vi "op_theremin_main.vi"() -> ()   [LabVIEW 2018]
uses:
  op_theremin_state_defining_enum.ctl
  sig_processing_state_defining_enum.ctl
panel:
  in  "Frequency 2":dbl(knob) min=0.0 max=20000.0 scale=0.0..20000.0
  in  "Frequency":dbl(knob) min=0.0 max=20000.0 scale=0.0..20000.0
  in  "Vertical Pointer Slide":dbl(slide) scale=0.0..10.0
  in  "Frequency":dbl(slide)=20.0 min=0.0 max=20000.0 scale=0.0..20000.0
  in  "Stop":bool
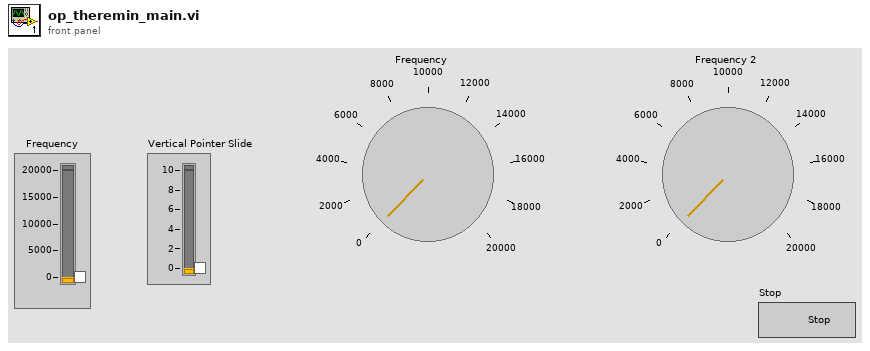
[diagram p1: front panel]
types:
  T1 = typedef "op_theremin_state_defining_enum.ctl" = enum16{"INIT", "SHDN", "RUN"}
  T2 = typedef "sig_processing_state_defining_enum.ctl" = enum16{"Coerce", "Scale", "Offset", "Norm"}
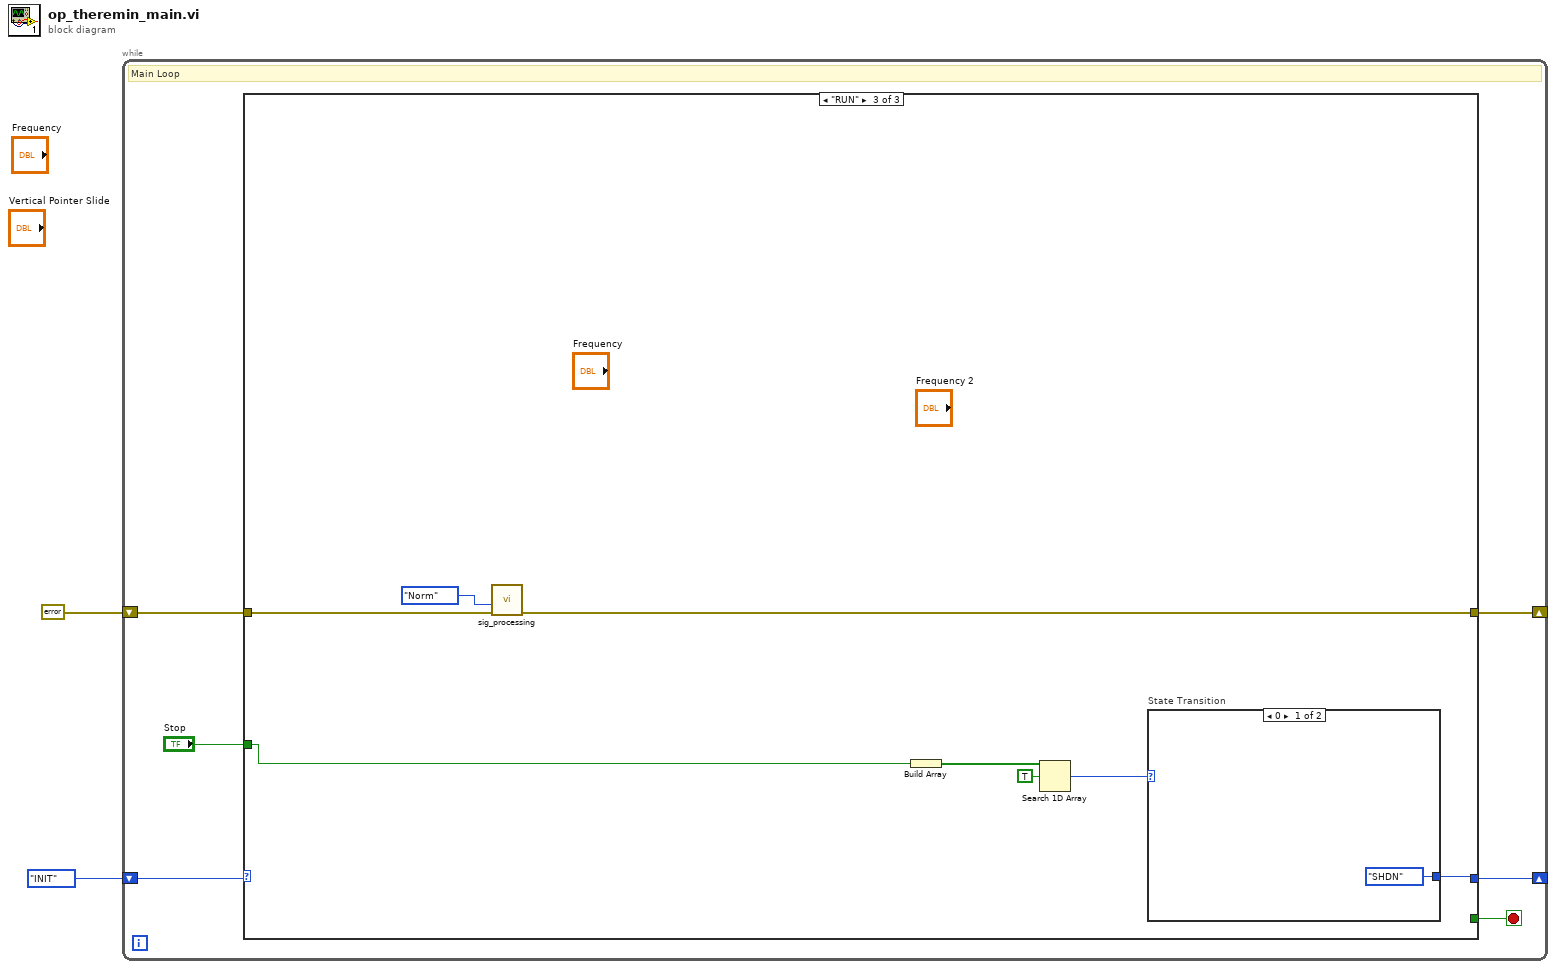
[diagram p0: block diagram]
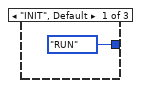
[diagram p2: hidden frame]
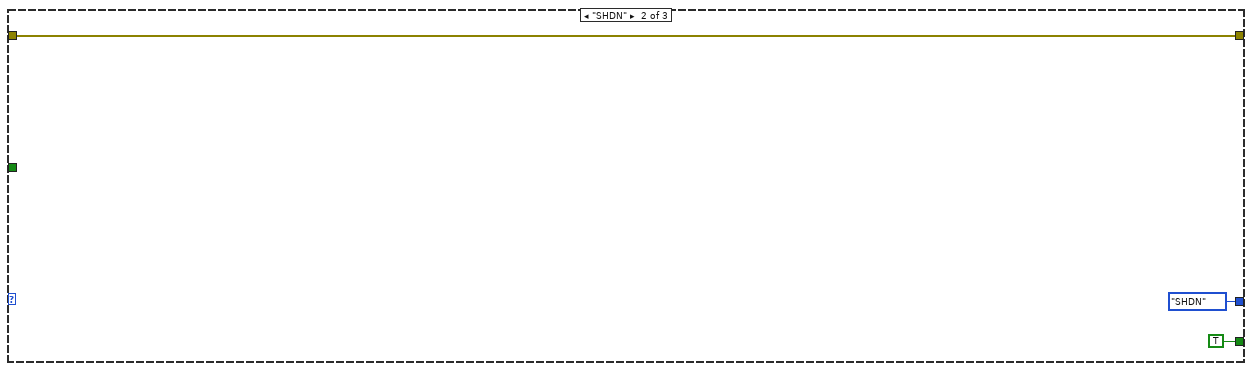
[diagram p3: hidden frame]
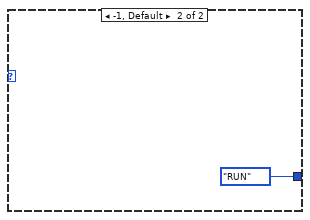
[diagram p4: hidden frame]
diagram:
  n1 = while {
    shift-right: [w6] -> _
    shift-left: op_theremin_state_defining_enum."INIT" -> [w7]
    shift-right: [w3] -> _
    shift-left: errorcluster {"status"=FALSE, "code"=0, "source"=""} ("error constant") -> [w4]
    stop <- w8 stop-if-true
    # "Main Loop"
    n2 = case shown="\"RUN\"" w7 {
      tunnel: [_ TRUE _] -> w8
      tunnel: [op_theremin_state_defining_enum."RUN" op_theremin_state_defining_enum."SHDN" w18] -> w6
      tunnel: "Stop" -> [_ _ w17]
      tunnel: w4 -> [_ w11 w15]
      tunnel: [_ w11 w14] -> w3
      frame "INIT", Default {
      }
      frame "SHDN" {
      }
      frame "RUN" {
        n3 = call "sig_processing.vi"("error in (no error)"=w15, "Operation"=sig_processing_state_defining_enum."Norm") -> ("error out"=w14:errorcluster)  [unwired: 8 in, 1 out]
        n4 = Build Array(w17) -> (w16:bool[])
        n5 = Search 1D Array(1D array=w16, element=TRUE) -> (index of element=w19:i32)  [unwired: 1 in]
        n6 = case "State Transition" shown="0" w19 {
          tunnel: [op_theremin_state_defining_enum."SHDN" op_theremin_state_defining_enum."RUN"] -> w18
          frame 0 {
            # "State Transition"
          }
          frame -1, Default {
          }
        }
      }
    }
  }
